vi "疫苗信息录入.vi"(5 "connection":T2) -> (0 "途径地点":i32, 1 "运输路线":cluster{"城市":string, bool}[](array[cluster]), 2 "疫苗信息":T1[](array[typedef]) {"生产日期" format="%<%Y/%m/%d>T"})   [LabVIEW 2018]
uses:
  <vilib>/addons/database/Connection.llb/Conn ObjectReference.ctl
  <vilib>/addons/database/Connection.llb/DB Tools Open Connec (Path).vi
  <vilib>/addons/database/NI_Database_API.lvlib
panel:
  out "error out":errorcluster
  in  "运输点（城市）":string
  in  "疫苗功能":string="预防virus感染"
  in  "是否检验合格":bool=TRUE
  in  "生产负责人":string="DOCH"
  in  "生产地":string="XZ"
  in  "生产日期":timestamp=timestamp(3639467727.664838 s since 1904-01-01) format="%<%Y/%m/%d>T"
  in  "生产厂家":string="JSFMF"
  in  "是否为第一类疫苗":bool=TRUE
  in  "疫苗名":string="ANTIVIRUS"
  in  "结束":bool
  in  "inextc":bool
  in  "stopvi":bool
  in  "Inextv":bool
  in  "开始":bool
  # "疫苗信息及运输路径设置"
  # "本界面用于疫苗信息输入，点击”开始输入“开始输入信息，每输入一种疫苗信息点击“写入疫苗信息”结束，输入所有的疫苗信息后按“结束疫苗信息输入“结束，进入运输路径输入，设置本次运输的出发点和目标点以及沿途经过的城市点。不输入无法结束，输入结束后按结束按钮退出本次信息录入\n开始输入按钮只可以点一次\n在输入运输路径后不可以再进行疫苗信息录入"
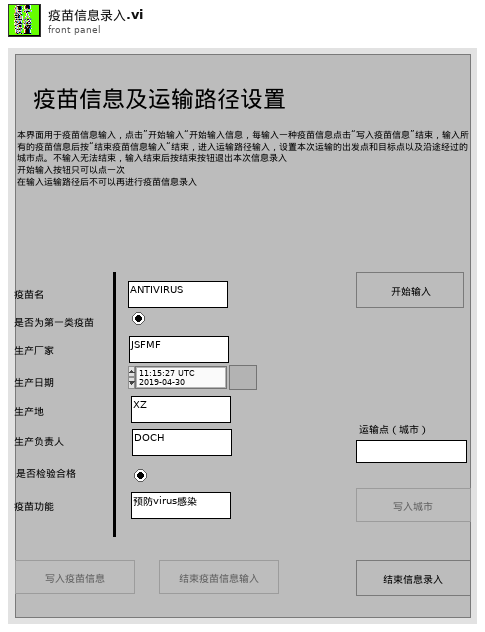
[diagram p1: front panel]
types:
  T1 = typedef "疫苗信息.ctl" = cluster{"疫苗名":string, "疫苗编号":i32, "疫苗类型":string, "生产厂家":string, "生产日期":timestamp, "生产地":string, "生产负责人":string, "是否合格":string, "疫苗功能":string}
  T2 = typedef "NI_Database_API.lvlib/Conn ObjectReference.ctl" = refnum<k1>
  T3 = enum8{"Enabled", "Disabled", "Disabled and Grayed Out"}
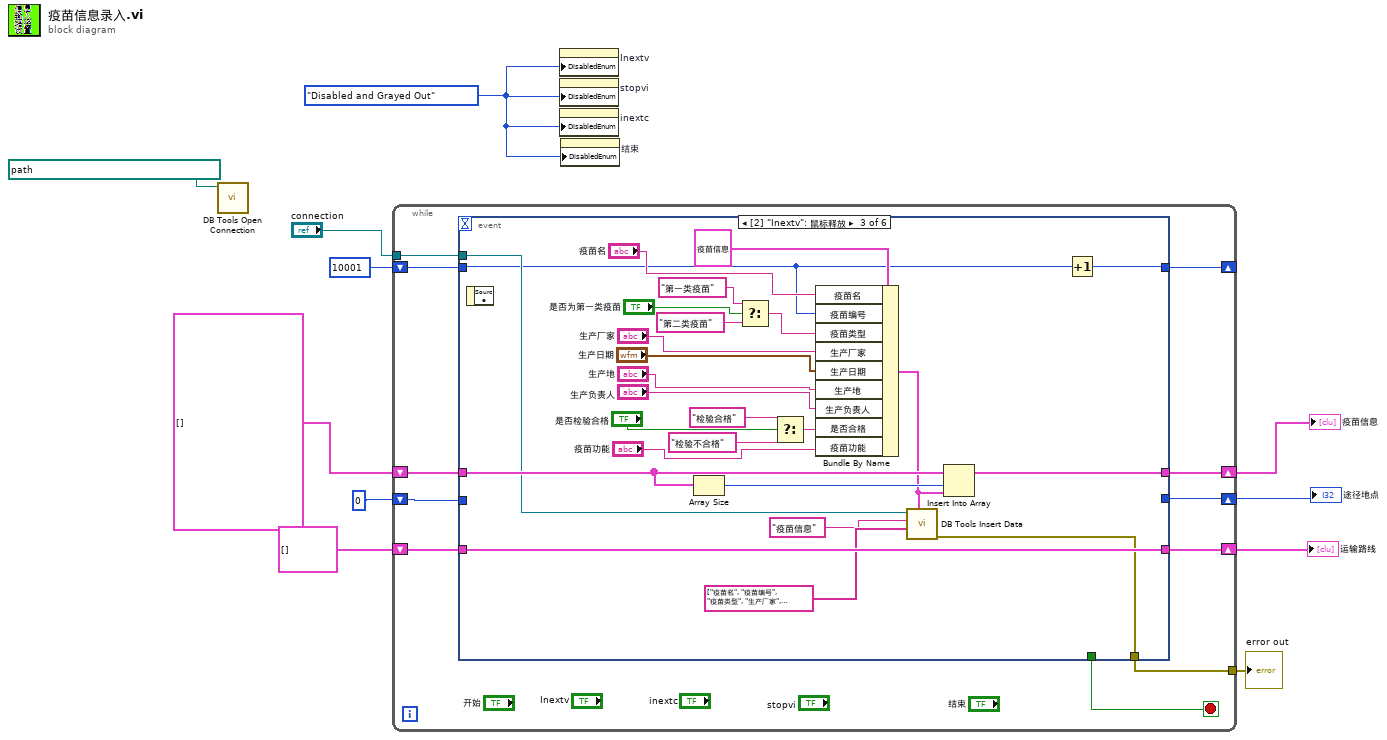
[diagram p0: block diagram]
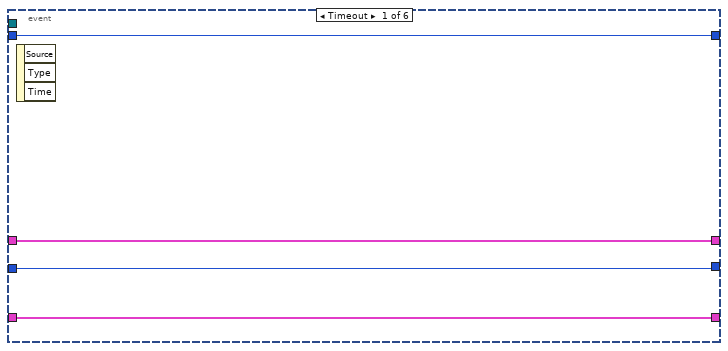
[diagram p2: hidden frame]
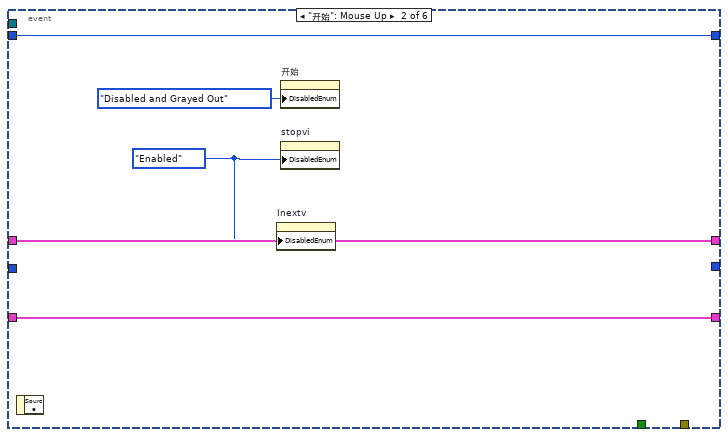
[diagram p3: hidden frame]
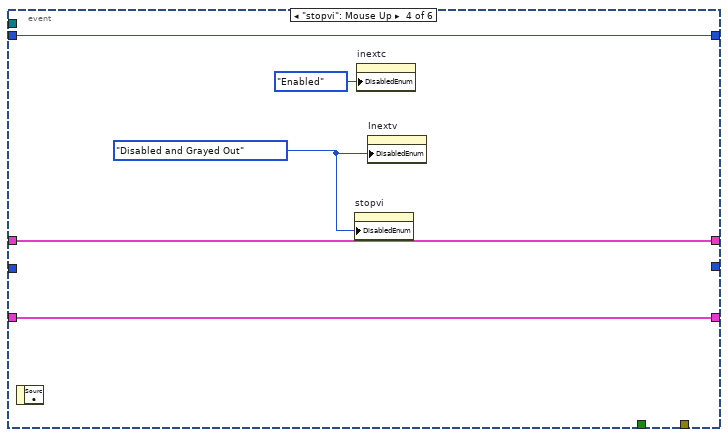
[diagram p4: hidden frame]
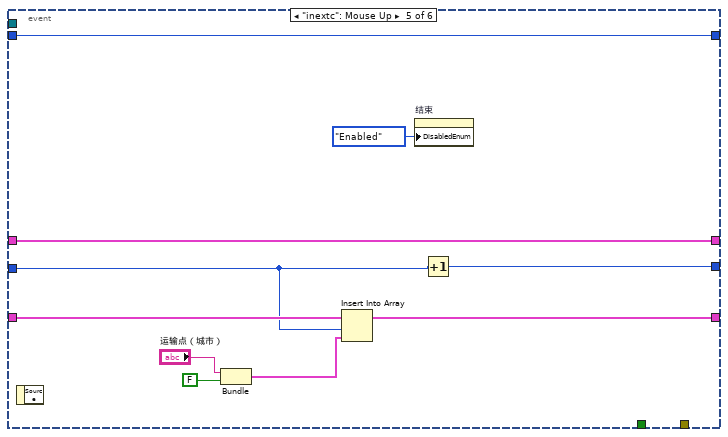
[diagram p5: hidden frame]
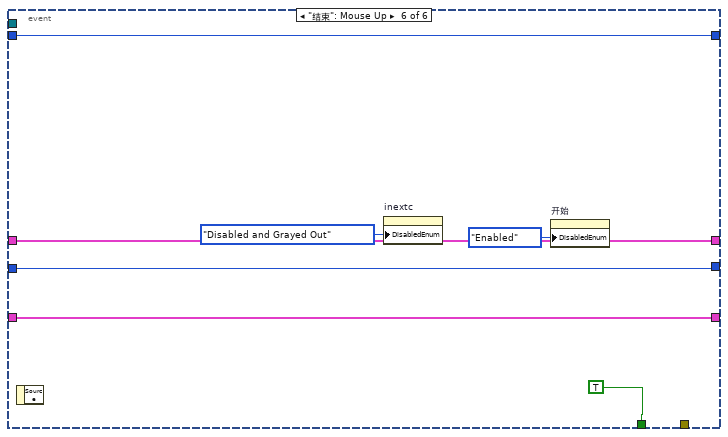
[diagram p6: hidden frame]
diagram:
  w4 = T3."Disabled and Grayed Out" ("禁用")
  n1 = call-poly <vilib>:"DB Tools Open Connection.vi"("connection information"=path "D:/2019毕业设计/Code/GPData.udl" ("路径")) -> ()  [unwired: 7 in, 2 out]
  n2 = while {
    shift-right: [w22] -> _
    shift-left: 10001 -> [w21]
    shift-right: [w20] -> w8
    shift-left: T1[] [] -> [w19]
    shift-right: [w18] -> w7
    shift-left: cluster{string, bool}[] [] -> [w17]
    shift-right: [w15] -> w3
    shift-left: 0 -> [w16]
    tunnel: "connection" -> [w14]
    tunnel: [w12] -> w2
    stop <- w13 stop-if-true
    n3 = event shown="[2] \"Inextv\": 鼠标释放" {
      selector: _ -> [_ _ _ _ _ _]
      dyn-events: _ -> [_ _ _ _ _ _]
      timeout: _ -> [_ _ _ _ _ _]
      tunnel: [w26 w31 w57 w62 w72 w79] -> w22
      tunnel: w21 -> [w26 w31 w42 w62 w72 w79]
      tunnel: [w25 w30 w55 w61 w71 w78] -> w20
      tunnel: w19 -> [w25 w30 w53 w61 w71 w78]
      tunnel: [w23 w29 w54 w60 w69 w76] -> w18
      tunnel: w17 -> [w23 w29 w54 w60 w70 w76]
      tunnel: w16 -> [w24 _ _ _ w68 w77]
      tunnel: [w24 _ _ _ w67 w77] -> w15
      tunnel: [_ _ _ _ _ TRUE] -> w13
      tunnel: w14 -> [_ _ w52 _ _ _]
      tunnel: [_ _ w49 _ _ _] -> w12
      event Timeout {
        n4 = event-data() -> ()  [unwired: 1 in, 3 out]
      }
      event "开始": Mouse Up {
        w27 = T3."Enabled" ("禁用")
        n5 = event-data() -> ()  [unwired: 1 in, 1 out]
        n6 = property on="Inextv" class="Bool (严格)"("DisabledEnum"=w27) -> ()  [unwired: 2 in, 2 out]
        n7 = property on="开始" class="Bool (严格)"("DisabledEnum"=T3."Disabled and Grayed Out" ("禁用")) -> ()  [unwired: 2 in, 2 out]
        n8 = property on="stopvi" class="Bool (严格)"("DisabledEnum"=w27) -> ()  [unwired: 2 in, 2 out]
      }
      event "Inextv": Mouse Up {
        n9 = event-data() -> ()  [unwired: 1 in, 1 out]
        n10 = Array Size(array=w53) -> (size(s)=w56:i32)
        n11 = Select(t="第一类疫苗", s="是否为第一类疫苗", f="第二类疫苗") -> (s? t:f=w40:string)
        n12 = Select(t="检验合格", s="是否检验合格", f="检验不合格") -> (s? t:f=w36:string)
        n13 = Bundle By Name(cluster=T1 {"疫苗名"="", "疫苗编号"=0, "疫苗类型"="", "生产厂家"="", "生产日期"=timestamp(0 s since 1904-01-01), "生产地"="", "生产负责人"="", "是否合格"="", "疫苗功能"=""} ("疫苗信息"), "疫苗名"="疫苗名", "疫苗编号"=w42, "疫苗类型"=w40, "生产厂家"="生产厂家", "生产日期"="生产日期", "生产地"="生产地", "生产负责人"="生产负责人", "是否合格"=w36, "疫苗功能"="疫苗功能") -> (w32:T1)
        n14 = call <vilib>:"DB Tools Insert Data.vi"("data"=w32, "columns"=string[] ["疫苗名", "疫苗编号", "疫苗类型", "生产厂家", "生产日期", "生产地", "生产负责人", "检验结果", "疫苗功能"], "table"="疫苗信息", "connection reference"=w52) -> ("error out"=w49:errorcluster)  [unwired: 6 in, 1 out]
        n15 = Insert Into Array(array=w53, index=w56, new element=w32) -> (w55:T1[])
        n16 = Increment(x=w42) -> (x+1=w57:i32)
      }
      event "stopvi": Mouse Up {
        w58 = T3."Disabled and Grayed Out" ("禁用")
        n17 = event-data() -> ()  [unwired: 1 in, 1 out]
        n18 = property on="stopvi" class="Bool (严格)"("DisabledEnum"=w58) -> ()  [unwired: 2 in, 2 out]
        n19 = property on="inextc" class="Bool (严格)"("DisabledEnum"=T3."Enabled" ("禁用")) -> ()  [unwired: 2 in, 2 out]
        n20 = property on="Inextv" class="Bool (严格)"("DisabledEnum"=w58) -> ()  [unwired: 2 in, 2 out]
      }
      event "inextc": Mouse Up {
        n21 = event-data() -> ()  [unwired: 1 in, 1 out]
        n22 = Bundle("运输点（城市）"="运输点（城市）", FALSE) -> (w64:cluster{"运输点（城市）":string, bool})  [unwired: 1 in]
        n23 = Insert Into Array(array=w70, index=w68, new element=w64) -> (w69:cluster{string, bool}[])
        n24 = property on="结束" class="Bool (严格)"("DisabledEnum"=T3."Enabled" ("禁用")) -> ()  [unwired: 2 in, 2 out]
        n25 = Increment(x=w68) -> (x+1=w67:i32)
      }
      event "结束": Mouse Up {
        n26 = event-data() -> ()  [unwired: 1 in, 1 out]
        n27 = property on="inextc" class="Bool (严格)"("DisabledEnum"=T3."Disabled and Grayed Out" ("禁用")) -> ()  [unwired: 2 in, 2 out]
        n28 = property on="开始" class="Bool (严格)"("DisabledEnum"=T3."Enabled" ("禁用")) -> ()  [unwired: 2 in, 2 out]
      }
    }
  }
  "疫苗信息" <- w8
  "运输路线" <- w7
  "途径地点" <- w3
  "error out" <- w2
  n29 = property on="Inextv" class="Bool (严格)"("DisabledEnum"=w4) -> ()  [unwired: 2 in, 2 out]
  n30 = property on="stopvi" class="Bool (严格)"("DisabledEnum"=w4) -> ()  [unwired: 2 in, 2 out]
  n31 = property on="inextc" class="Bool (严格)"("DisabledEnum"=w4) -> ()  [unwired: 2 in, 2 out]
  n32 = property on="结束" class="Bool (严格)"("DisabledEnum"=w4) -> ()  [unwired: 2 in, 2 out]
